vi "Buttons And Axis To Controller.vi"(6 "All Axis":T13, 7 "Buttons":T15) -> (1 "Controller":T1={"A Button"=FALSE, "B Button"=FALSE, "X Button"=FALSE, "Y Button"=FALSE, "Left Bumper"=FALSE, "Right Bumper"=FALSE, "View Button"=FALSE, "Menu Button"=FALSE, "Left Stick"={[], []}, "Right Stick"={[], []}, "Trigger"=0, "D-Pad"=5} {"Trigger" scale=32767.0..-32768.0})   [LabVIEW 2011, in "LMH-Xbox-One-Controller.lvlib"]
uses:
  LMH-Xbox-One-Controller.lvlib
  Type Defs/Indicators/All Buttons Visual.ctl
  Type Defs/Indicators/A.ctl
  Type Defs/Indicators/B.ctl
  Type Defs/Indicators/X.ctl
  Type Defs/Indicators/Y.ctl
  Type Defs/Indicators/Left Bumper.ctl
  Type Defs/Indicators/Right Bumper.ctl
  Type Defs/Indicators/View.ctl
  Type Defs/Indicators/Menu.ctl
  Type Defs/Indicators/Thumbstick.ctl
  Type Defs/Indicators/All Axis Data.ctl
  Type Defs/Indicators/DPad Enum.ctl
  Type Defs/Indicators/Controller.ctl
  Type Defs/Indicators/Thumbstick_Analog.ctl
  Type Defs/Indicators/Slider.ctl
  Type Defs/Indicators/DPad.ctl
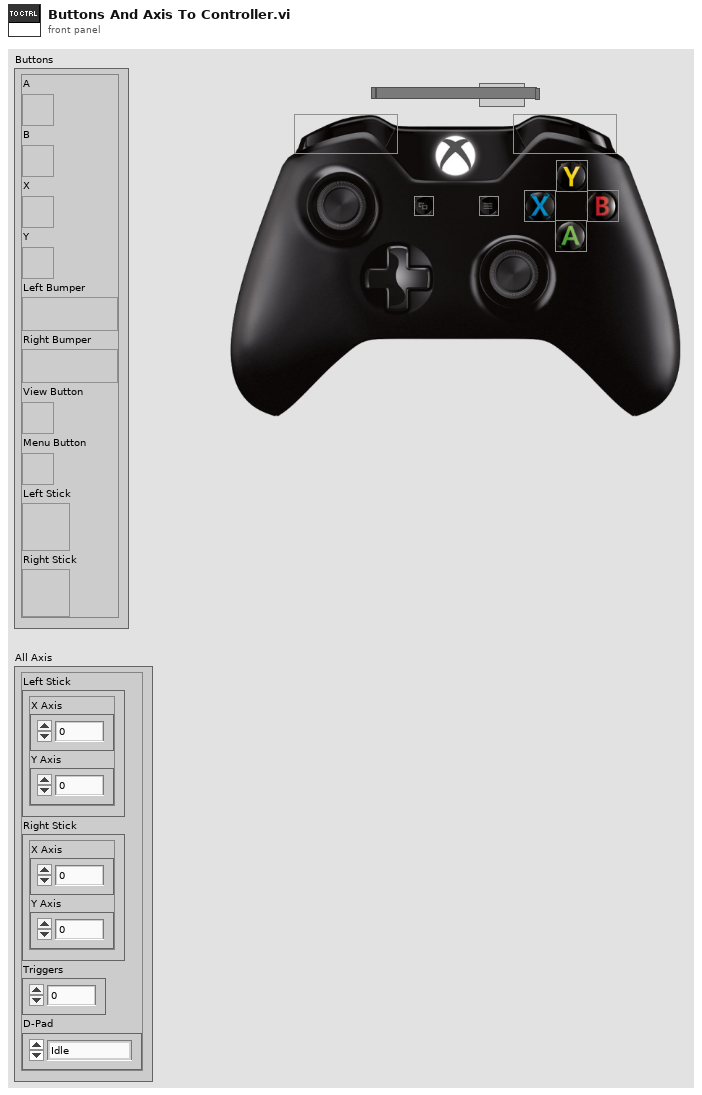
[diagram p1: front panel]
types:
  T1 = typedef "LMH-Xbox-One-Controller.lvlib/Controller.ctl" = cluster{"A Button":T2, "B Button":T3, "X Button":T4, "Y Button":T5, "Left Bumper":T6, "Right Bumper":T7, "View Button":T8, "Menu Button":T9, "Left Stick":T10, "Right Stick":T10, "Trigger":T11, "D-Pad":T12}
  T2 = typedef "LMH-Xbox-One-Controller.lvlib/A.ctl" = bool
  T3 = typedef "LMH-Xbox-One-Controller.lvlib/B.ctl" = bool
  T4 = typedef "LMH-Xbox-One-Controller.lvlib/X.ctl" = bool
  T5 = typedef "LMH-Xbox-One-Controller.lvlib/Y.ctl" = bool
  T6 = typedef "LMH-Xbox-One-Controller.lvlib/Left Bumper.ctl" = bool
  T7 = typedef "LMH-Xbox-One-Controller.lvlib/Right Bumper.ctl" = bool
  T8 = typedef "LMH-Xbox-One-Controller.lvlib/View.ctl" = bool
  T9 = typedef "LMH-Xbox-One-Controller.lvlib/Menu.ctl" = bool
  T10 = typedef "LMH-Xbox-One-Controller.lvlib/Thumbstick_Analog.ctl" = cluster{i32[], i32[]}
  T11 = typedef "LMH-Xbox-One-Controller.lvlib/Slider.ctl" = i32
  T12 = typedef "LMH-Xbox-One-Controller.lvlib/DPad.ctl" = u16
  T13 = typedef "LMH-Xbox-One-Controller.lvlib/All Axis Data.ctl" = cluster{"Left Stick":cluster{"X Axis":i32, "Y Axis":i32}, "Right Stick":cluster{"X Axis":i32, "Y Axis":i32}, "Triggers":i32, "D-Pad":T14}
  T14 = typedef "LMH-Xbox-One-Controller.lvlib/DPad Enum.ctl" = enum16{"Idle", "Up", "Up / Right", "Right", "Down / Right", "Down", "Down / Left", "Left", "Up / Left"}
  T15 = typedef "LMH-Xbox-One-Controller.lvlib/All Buttons Visual.ctl" = cluster{"A":T2, "B":T3, "X":T4, "Y":T5, "Left Bumper":T6, "Right Bumper":T7, "View Button":T8, "Menu Button":T9, "Left Stick":T16, "Right Stick":T16}
  T16 = typedef "LMH-Xbox-One-Controller.lvlib/Thumbstick.ctl" = bool
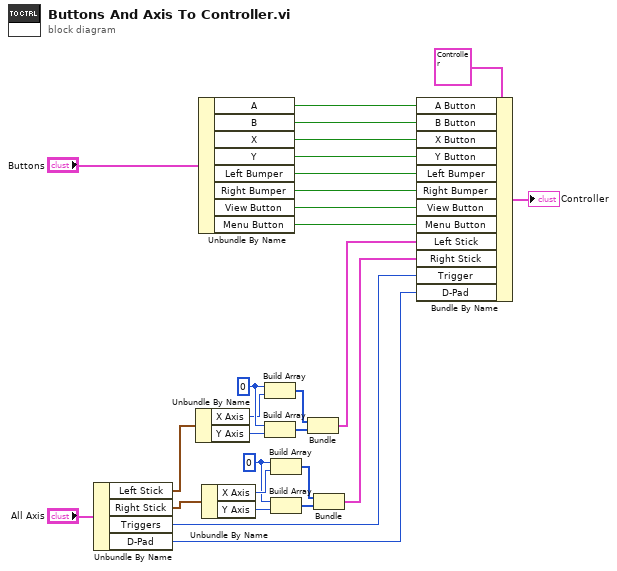
[diagram p0: block diagram]
diagram:
  w7 = 0 ("element")
  w14 = 0 ("element")
  n1 = Unbundle By Name("All Axis") -> ("Left Stick"=w13:cluster{"X Axis":i32, "Y Axis":i32}, "Right Stick"=w4:cluster{"X Axis":i32, "Y Axis":i32}, "Triggers"=w2:i32, "D-Pad"=w1:T14)
  n2 = Unbundle By Name(w13) -> ("X Axis"=w12:i32, "Y Axis"=w11:i32)
  n3 = Unbundle By Name("Buttons") -> ("A"=w24:T2, "B"=w23:T3, "X"=w22:T4, "Y"=w21:T5, "Left Bumper"=w20:T6, "Right Bumper"=w19:T7, "View Button"=w18:T8, "Menu Button"=w17:T9)
  n4 = Unbundle By Name(w4) -> ("X Axis"=w8:i32, "Y Axis"=w9:i32)
  n5 = Build Array(w14, w12) -> (w16:i32[])
  n6 = Build Array(w14, w11) -> (w15:i32[])
  n7 = Build Array(w7, w8) -> (w5:i32[])
  n8 = Build Array(w7, w9) -> (w6:i32[])
  n9 = Bundle(w16, w15) -> (w10:cluster{i32[], i32[]})  [unwired: 1 in]
  n10 = Bundle(w5, w6) -> (w3:cluster{i32[], i32[]})  [unwired: 1 in]
  n11 = Bundle By Name(cluster=T1 {"A Button"=FALSE, "B Button"=FALSE, "X Button"=FALSE, "Y Button"=FALSE, "Left Bumper"=FALSE, "Right Bumper"=FALSE, "View Button"=FALSE, "Menu Button"=FALSE, "Left Stick"={[], []}, "Right Stick"={[], []}, "Trigger"=0, "D-Pad"=5} ("Controller"), "A Button"=w24, "B Button"=w23, "X Button"=w22, "Y Button"=w21, "Left Bumper"=w20, "Right Bumper"=w19, "View Button"=w18, "Menu Button"=w17, "Left Stick"=w10, "Right Stick"=w3, "Trigger"=w2, "D-Pad"=w1) -> (→"Controller":T1)
